vi "amc_Send Message over UDP.vi"(8 "error in":errorcluster, 11 "Message":T1) -> (0 "error out":errorcluster, 1 "Receiver Host":string, 2 "Message XML String":string)   [LabVIEW 2013, in "main.lvlib" / "TLB_Dependencies.lvlib"]
uses:
  TLB_Dependencies.lvlib
  amc_Message.ctl
  <vilib>/FTP/util/Keyed Array.ctl
  <vilib>/FTP/NI_FTP.lvlib
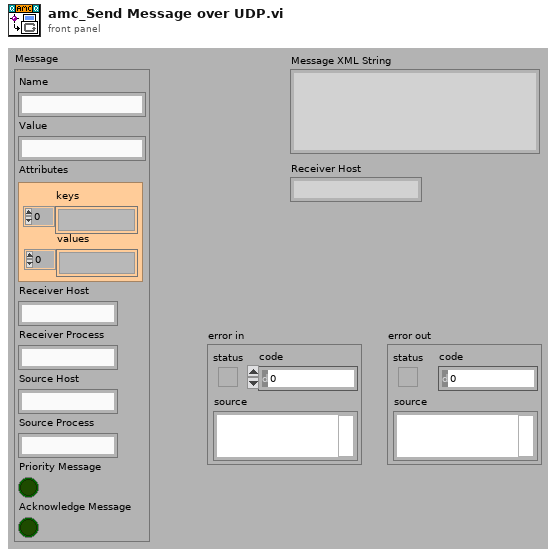
[diagram p1: front panel]
types:
  T1 = typedef "main.lvlib/TLB_Dependencies.lvlib/amc_Message.ctl" = cluster{"Name":string, "Value":string, "Attributes":T2, "Receiver Host":string, "Receiver Process":string, "Source Host":string, "Source Process":string, "Priority Message":bool, "Acknowledge Message":bool}
  T2 = typedef "NI_FTP.lvlib/Keyed Array.ctl" = cluster{"keys":string[], "values":string[]}
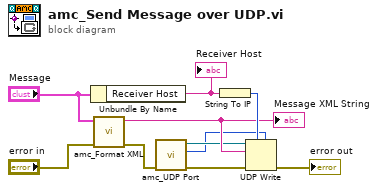
[diagram p0: block diagram]
diagram:
  n1 = Unbundle By Name("Message") -> ("Receiver Host"=w8:string)
  "Receiver Host" <- w8
  n2 = call "amc_Format XML.vi"("error in (no error)"="error in", "Message"="Message") -> ("error out"=w1:errorcluster, "Message XML String"=w9:string)  [unwired: 8 out]
  "Message XML String" <- w9
  n3 = call "amc_UDP Port.vi"("error in (no error)"=w1) -> ("error out"=w6:errorcluster, "UDP Port"=w5:u16, "UDP Port Ref"=w7:refnum<k16>)  [unwired: 2 in, 6 out]
  n4 = String To IP(1:w8) -> (0:w10:u32)
  n5 = UDP Write(address=w10, port or service name=w5, connection ID=w7, data in=w9, 8:w6) -> (error out=→"error out":errorcluster)  [unwired: 2 out]
